vi "Table Number 2 Dataset Source.vi"(4 "Rigid Connection":bool, 5 "Table Number":i32, 6 "Number of\nLBCBs":T2) -> (0 "Invalid":bool, 1 "Dataset Source":T1, 2 "IsCommand":bool)   [LabVIEW 2009]
uses:
  Data Access Objects/Application/Number Of LBCBs.ctl
  Global Data/Transactions/Dataset Source.ctl
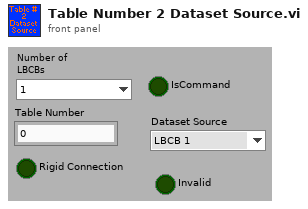
[diagram p1: front panel]
types:
  T1 = typedef "Dataset Source.ctl" = enum16{"LBCB 1", "LBCB 2", "Combined", "External Sensors"}
  T2 = typedef "Number Of LBCBs.ctl" = enum16{"1", "2"}
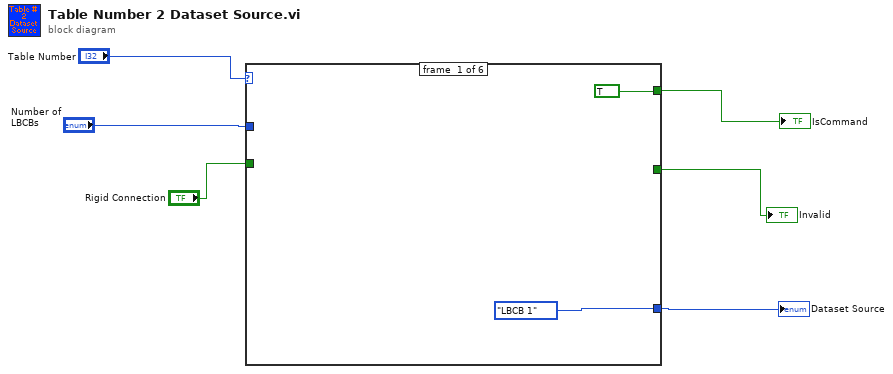
[diagram p0: block diagram]
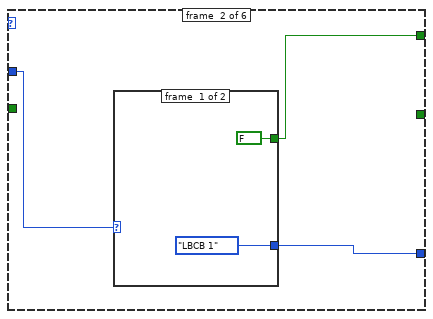
[diagram p2: hidden frame]
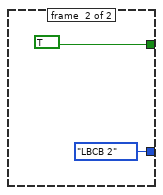
[diagram p3: hidden frame]
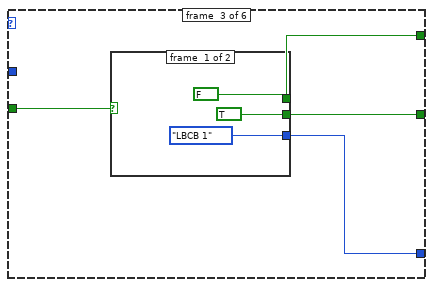
[diagram p4: hidden frame]
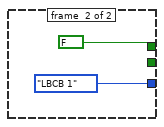
[diagram p5: hidden frame]
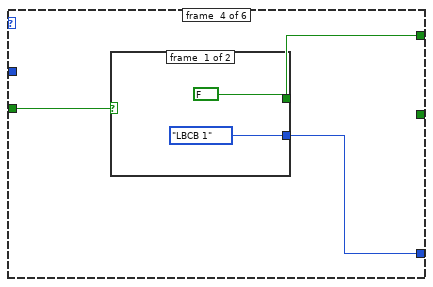
[diagram p6: hidden frame]
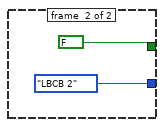
[diagram p7: hidden frame]
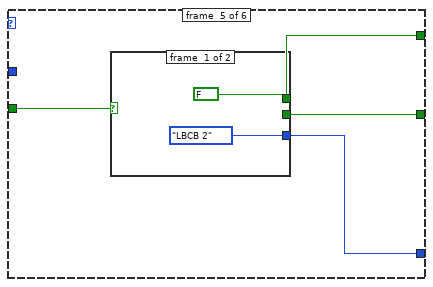
[diagram p8: hidden frame]
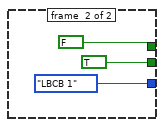
[diagram p9: hidden frame]
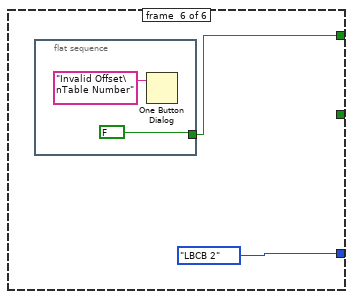
[diagram p10: hidden frame]
diagram:
  n1 = case shown="5, Default" "Table Number" {
    tunnel: [Dataset_Source."LBCB 1" ("Dataset Source") w11 w19 w27 w35 Dataset_Source."LBCB 2" ("Dataset Source")] -> w4
    tunnel: [TRUE w9 w17 w25 w33 w41] -> w5
    tunnel: "Number of\nLBCBs" -> [_ w10 _ _ _ _]
    tunnel: "Rigid Connection" -> [_ _ w18 w26 w34 _]
    tunnel: [_ _ w16 _ w32 _] -> w1
    frame #0 {
    }
    frame #1 {
      n2 = case shown="\"2\"" w10 {
        tunnel: [Dataset_Source."LBCB 1" ("Dataset Source") Dataset_Source."LBCB 2" ("Dataset Source")] -> w11
        tunnel: [FALSE TRUE] -> w9
        frame #0 {
        }
        frame #1 {
        }
      }
    }
    frame #2 {
      n3 = case shown="False" w18 {
        tunnel: [Dataset_Source."LBCB 1" ("Dataset Source") Dataset_Source."LBCB 1" ("Dataset Source")] -> w19
        tunnel: [FALSE FALSE] -> w17
        tunnel: [TRUE _] -> w16
        frame #0 {
        }
        frame #1 {
        }
      }
    }
    frame #3 {
      n4 = case shown="False" w26 {
        tunnel: [Dataset_Source."LBCB 1" ("Dataset Source") Dataset_Source."LBCB 2" ("Dataset Source")] -> w27
        tunnel: [FALSE FALSE] -> w25
        frame #0 {
        }
        frame #1 {
        }
      }
    }
    frame #4 {
      n5 = case shown="False" w34 {
        tunnel: [Dataset_Source."LBCB 2" ("Dataset Source") Dataset_Source."LBCB 1" ("Dataset Source")] -> w35
        tunnel: [FALSE FALSE] -> w33
        tunnel: [_ TRUE] -> w32
        frame #0 {
        }
        frame #1 {
        }
      }
    }
    frame #5 {
      n6 = flat-sequence {
        tunnel: [FALSE] -> w41
        frame #0 {
          n7 = One Button Dialog(message="Invalid Offset\nTable Number") -> ()  [unwired: 1 in, 1 out]
        }
      }
    }
  }
  "IsCommand" <- w5
  "Dataset Source" <- w4
  "Invalid" <- w1
